vi "EXPRES Format Lamp Status Message.vi"(8 "error in":errorcluster, 10 "Lamps":T1) -> (0 "error out":errorcluster, 2 "JSON string":string)   [LabVIEW 2016]
uses:
  Controls/All Lamps.ctl
  Controls/Lamp Data.ctl
  Controls/Lamp Status Message.ctl
  Controls/Messages/Lamp Message Struct.ctl
  Libs/Messages.lvlib
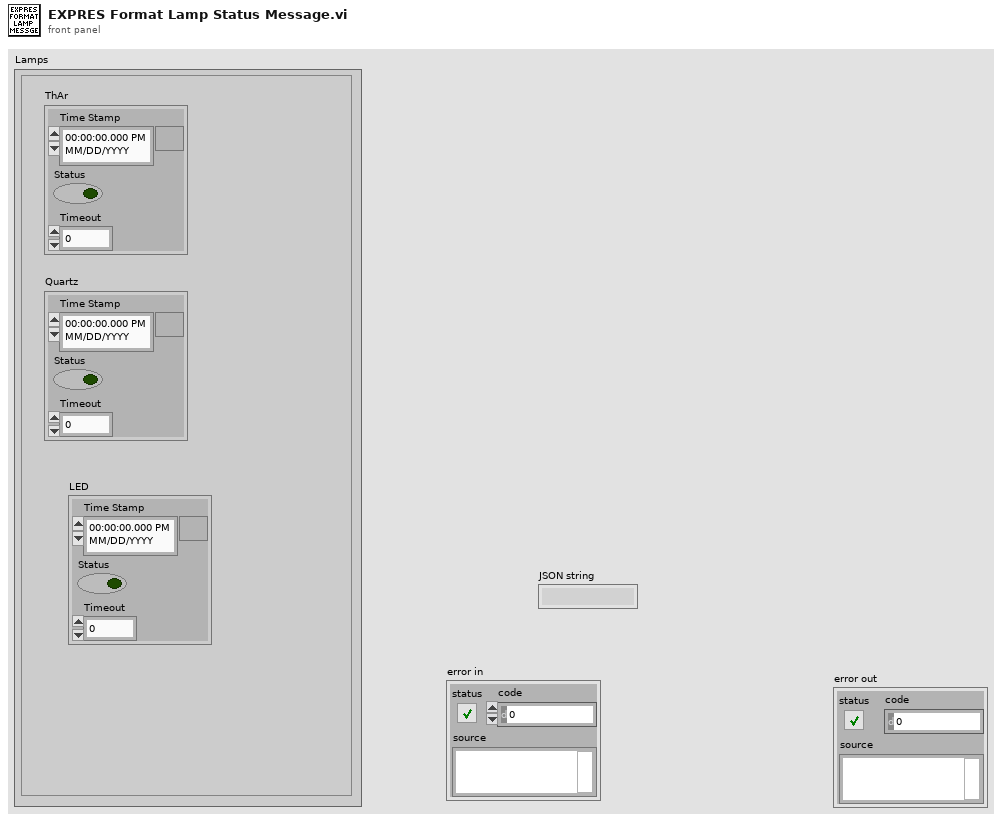
[diagram p1: front panel]
types:
  T1 = typedef "All Lamps.ctl" = cluster{"Lamp":T2, "Quartz":T2, "LED":T2}
  T2 = typedef "Lamp Data.ctl" = cluster{"Time Stamp":timestamp, "Status":bool, "Timeout":dbl}
  T3 = typedef "Messages.lvlib/Lamp Status Message.ctl" = cluster{"ThAr":T4, "Quartz":T4, "LED":T4}
  T4 = typedef "Messages.lvlib/Lamp Message Struct.ctl" = cluster{"time":string, "status":string, "timeout":string}
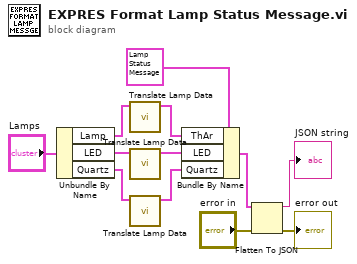
[diagram p0: block diagram]
diagram:
  n1 = Unbundle By Name("Lamps") -> ("Lamp"=w6:T2, "LED"=w7:T2, "Quartz"=w8:T2)
  n2 = call "Translate Lamp Data.vi"("Lamp"=w6) -> ("output lamp message"=w4:T4)  [unwired: 10 in]
  n3 = call "Translate Lamp Data.vi"("Lamp"=w7) -> ("output lamp message"=w3:T4)  [unwired: 10 in]
  n4 = call "Translate Lamp Data.vi"("Lamp"=w8) -> ("output lamp message"=w2:T4)  [unwired: 10 in]
  n5 = Bundle By Name(cluster=T3 {"ThAr"={"time"="", "status"="", "timeout"=""}, "Quartz"={"time"="", "status"="", "timeout"=""}, "LED"={"time"="", "status"="", "timeout"=""}} ("Cluster"), "ThAr"=w4, "LED"=w3, "Quartz"=w2) -> (w1:T3)
  n6 = Flatten To JSON(anything=w1, error in (no error)="error in") -> (JSON string=→"JSON string":string, 11:→"error out":errorcluster)  [unwired: 1 in]
